vi "Source Output Enable.vi"(7 "Output (Off)":bool, 8 "error in (no error)":errorcluster, 9 "Channel (Channel A)":T1, 10 "Node In":string, 11 "VISA resource name":refnum<visa-resource-name>) -> (0 "error out":errorcluster, 2 "Node Out":string, 3 "VISA resource name out":refnum<visa-resource-name>, 4 "Command String":string)   [LabVIEW 2018, in "Keithley 2600 Series.lvlib"]
doc: "This VI turns the SMU output on or off.\n\n<b>Functions and Attributes Used</b>\nsmuX.source.output"
uses:
  Keithley 2600 Series.lvlib
  Channel.ctl
  GlobalVariables.vi
panel:
  # "(c) 2008 Keithley Instruments, Inc.  ALL RIGHTS RESERVED."
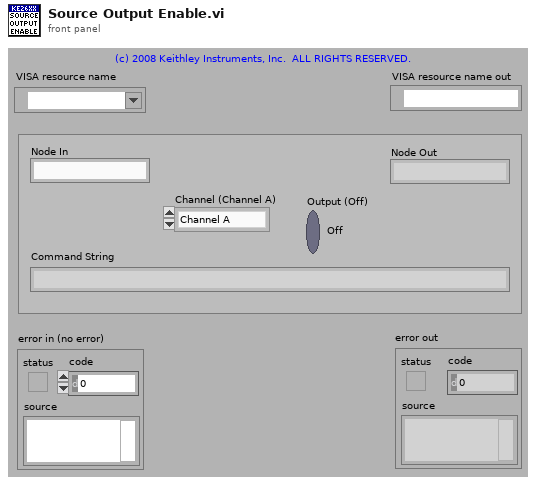
[diagram p1: front panel]
types:
  T1 = typedef "Keithley 2600 Series.lvlib/Channel.ctl" = enum32{"Channel A", "Channel B"}
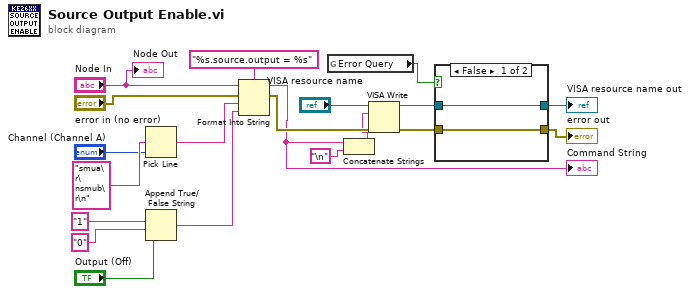
[diagram p0: block diagram]
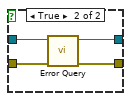
[diagram p2: hidden frame]
diagram:
  n1 = Pick Line(multi-line string="smua\r\nsmub\r\n" ("options"), line index="Channel (Channel A)") -> (output string=w8:string)  [unwired: 1 out]
  n2 = Append True/False String(1:"Output (Off)", 2:"0" ("false string"), 3:"1" ("true string")) -> (0:w7:string)  [unwired: 1 out]
  n3 = Format Into String(format string="%s.source.output = %s", initial string="Node In", error in="error in (no error)", w8, w7) -> (resulting string=w2:string, error out=w4:errorcluster)
  "Command String" <- w2
  n4 = global read "GlobalVariables.vi" "Error Query"() -> (w15:bool)
  n5 = Concatenate Strings(w2, "\n") -> (w1:string)
  n6 = VISA Write(VISA resource name="VISA resource name", write buffer=w1, error in (no error)=w4) -> (VISA resource name out=w14:refnum<visa-resource-name>, error out=w13:errorcluster)  [unwired: 1 out]
  n7 = case shown="False" w15 {
    tunnel: w14 -> [w22 w26]
    tunnel: w13 -> [w21 w25]
    tunnel: [w22 w24] -> w12
    tunnel: [w21 w23] -> w11
    frame False {
    }
    frame True {
      n8 = call "Error Query.vi"("error in (no error)"=w25, "VISA resource name"=w26) -> ("error out"=w23:errorcluster, "VISA resource name out"=w24:refnum<visa-resource-name>)  [unwired: 8 out]
    }
  }
  "VISA resource name out" <- w12
  "error out" <- w11
  "Node Out" <- "Node In"
